vi "galvo.scan.engine_grMD.vi"() -> ()   [LabVIEW 2012]
doc: "SciScan 1.2 160622"
uses:
  <vilib>/Utility/VariantDataType/Type.ctl
  Custom Controls/trigger enum.ctl
  hyperscope modules/hyperscope subVIs/Timebase and Trigger Routing.ctl
  Custom Controls/advanced settings inner tab CTL.ctl
  GFG/GFGbooleanGet.vi
  GFG/GFGnumericGet.vi
  GFG/GFGstringGet.vi
  GFG/GFGfpRefGet.vi
  <vilib>/DAQmx/read.llb/DAQmx Read (Analog 2D I16 NChan NSamp).vi
  GFG/GFG library.lvlib
  <vilib>/Utility/VariantDataType/VariantType.lvlib
panel:
  out "String 3":string
  in  "stop":bool
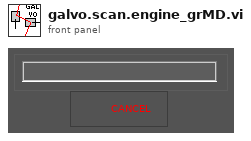
[diagram p1: front panel]
types:
  T1 = typedef "Timebase and Trigger Routing.ctl" = enum16{"Connect", "Disconnect all", "Disconnect Trigger"}
  T2 = typedef "trigger enum.ctl" = enum16{"legacy frame pulser PFI4", "continuous pulses", "single pulse", "trigger off"}
  T3 = enum32{"Invalid", "Default", "Floating", "Floating/Auto-Hide", "Modal"}
  T4 = enum32{"Invalid", "Standard", "Closed", "Hidden", "Minimized", "Maximized"}
  T5 = typedef "advanced settings inner tab CTL.ctl" = enum32{"arb. frames", "AO", "AI", "channels", "trigger", "Zstack data"}
  T6 = cluster{"NewVal":bool, "Event Registration Refnum":refnum<event-registration>}
  T7 = cluster{"WaveformChartRef":refnum<vi>, "DigitalRef":refnum<vi>, "ArrayRef":refnum<vi>, "TabControlRef":refnum<vi>, "EnumRef":refnum<vi>, "RingRef":refnum<vi>, "BooleanRef":refnum<vi>, "KnobRef":refnum<vi>, "SlideRef":refnum<vi>, "PathRef":refnum<vi>, "StringRef":refnum<vi>, "ComboBox":refnum<vi>, "WaveformGraphRef":refnum<vi>}
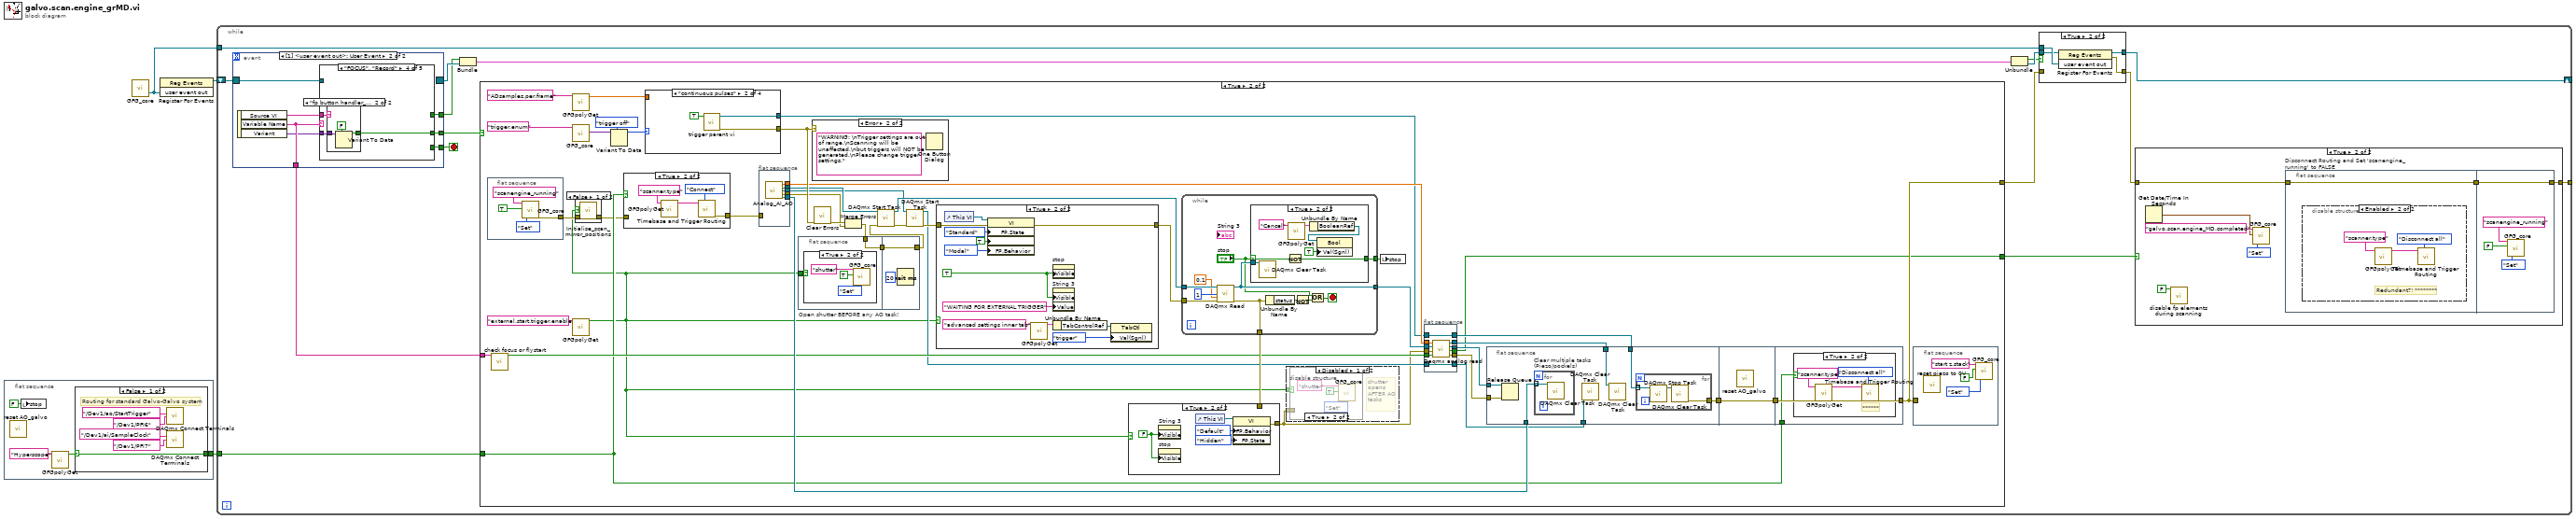
[diagram p0: block diagram]
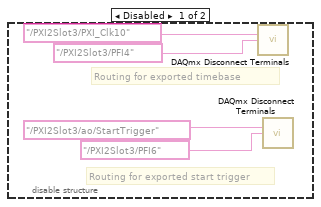
[diagram p5: hidden frame]
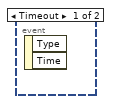
[diagram p6: hidden frame]
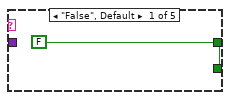
[diagram p7: hidden frame]
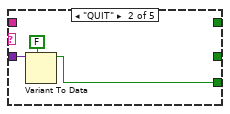
[diagram p8: hidden frame]
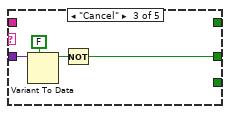
[diagram p9: hidden frame]
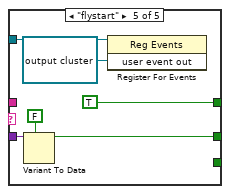
[diagram p11: hidden frame]
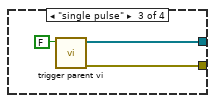
[diagram p20: hidden frame]
diagram:
  n1 = flat-sequence {
    tunnel: [w4] -> w1
    frame #0 {
      n2 = call "reset AO_galvo.vi"() -> ()  [unwired: 12 in]
      n3 = local write "stop"(FALSE ("stop")) -> ()
      n4 = call-poly "GFGpolyGet.vi"("Variable Name in"="Hyperscope") -> ("Boolean Value OUT"=w6:bool)  [unwired: 9 in, 1 out]
      n5 = case shown="False" w6 {
        selector: w6 -> [w9 w13]
        tunnel: [w9 w13] -> w4
        frame False {
          # "Routing for standard Galvo-Galvo system"
          n6 = call <vilib>:"DAQmx Connect Terminals.vi"("source terminal"=tag "/Dev1/ao/StartTrigger", "destination terminal"=tag "/Dev1/PFI6") -> ()  [unwired: 13 in, 1 out]
          n7 = call <vilib>:"DAQmx Connect Terminals.vi"("source terminal"=tag "/Dev1/ai/SampleClock", "destination terminal"=tag "/Dev1/PFI7") -> ()  [unwired: 13 in, 1 out]
        }
        frame True {
        }
      }
    }
  }
  n8 = call "GFG_core.vi"() -> ("user event out"=w2:refnum<user-event>)  [unwired: 13 in, 6 out]
  n9 = register-events(w2) -> (reference out=w3:refnum<event-registration>)  [unwired: 2 in, 1 out]
  n10 = while {
    tunnel: w2 -> [w26]
    shift-right: [w23] -> _
    shift-left: w3 -> [w27]
    tunnel: w1 -> [w16]
    tunnel: [w14] -> _
    stop <- w28 stop-if-true
    n11 = event shown="[1] <user event out>: User Event" {
      selector: w27 -> [_ w59]
      dyn-events: [_ _] -> w22
      timeout: _ -> [_ _]
      tunnel: [_ w62] -> w29
      tunnel: [_ w61] -> w28
      tunnel: [_ w58] -> w25
      tunnel: [_ w57] -> w21
      event Timeout {
        n12 = event-data() -> ()  [unwired: 1 in, 2 out]
      }
      event User Event {
        n13 = event-data() -> ("Source VI"=w60:string, "Variable Name"=w58:string, "Variant"=w56:variant)  [unwired: 1 in]
        n14 = case shown="\"FOCUS\", \"Record\"" w58 {
          tunnel: [w63 _ w67 w72 w80] -> w62
          tunnel: [w63 w64 _ _ _] -> w61
          tunnel: w56 -> [_ w66 w69 w73 w81]
          tunnel: w60 -> [_ _ _ w71 _]
          tunnel: w59 -> [_ _ _ _ w78]
          tunnel: [_ _ _ _ TRUE ("NewVal")] -> w57
          frame "False", Default {
            w63 = FALSE ("NewVal")
          }
          frame "QUIT" {
            n15 = Variant To Data(type=FALSE ("NewVal"), Variant=w66) -> (data=w64:bool)  [unwired: 1 in, 1 out]
          }
          frame "Cancel" {
            n16 = Variant To Data(type=FALSE ("NewVal"), Variant=w69) -> (data=w68:bool)  [unwired: 1 in, 1 out]
            n17 = Not(x=w68) -> (.not. x?=w67:bool)
          }
          frame "FOCUS", "Record" {
            n18 = case shown="\"fp button handler_crMD.vi\"" w71 {
              tunnel: w73 -> [_ w75]
              tunnel: [_ w74] -> w72
              frame "False", Default {
              }
              frame "fp button handler_crMD.vi" {
                n19 = Variant To Data(type=FALSE ("NewVal"), Variant=w75) -> (data=w74:bool)  [unwired: 1 in, 1 out]
              }
            }
          }
          frame "flystart" {
            n20 = Variant To Data(type=FALSE ("NewVal"), Variant=w81) -> (data=w80:bool)  [unwired: 1 in, 1 out]
            n21 = register-events(reference=w78, refnum<user-event> refnum ("user event out")) -> ()  [unwired: 1 in, 2 out]
          }
        }
      }
    }
    n22 = Bundle("NewVal"=w21, "Event Registration Refnum"=w22) -> (w20:T6)  [unwired: 1 in]
    n23 = case shown="True" w29 {
      tunnel: [_ w122] -> w24
      tunnel: w25 -> [_ w123]
      tunnel: [_ w95] -> w17
      tunnel: w16 -> [_ w90]
      frame False {
      }
      frame True {
        n24 = flat-sequence {
          tunnel: [w141] -> w85
          frame #0 {
            n25 = call "GFG_core.vi"("Variable Name in"="scanengine_running", "Variant in"=TRUE, "Action"=enum16{"Init", "Set", "Get"}."Set") -> ("error out"=w141:errorcluster)  [unwired: 10 in, 6 out]
          }
        }
        n26 = call "check focus or flystart.vi"("GFG variable name"=w123) -> ("Focus or flystart?"=w102:bool)  [unwired: 10 in]
        n27 = call-poly "GFGpolyGet.vi"("Variable Name in"="ADsamples.per.frame" ("Tag in")) -> ("Numeric"=w112:dbl)  [unwired: 8 in, 2 out]
        n28 = call "GFG_core.vi"("Variable Name in"="trigger.enum") -> ("Variant Out"=w118:variant)  [unwired: 12 in, 6 out]
        n29 = call-poly "GFGpolyGet.vi"("Variable Name in"="external.start.trigger.enable" ("Tag in")) -> ("Boolean Value OUT"=w83:bool)  [unwired: 9 in, 1 out]
        n30 = case shown="False" w83 {
          tunnel: w85 -> [w127 w128]
          tunnel: [w126 w128] -> w84
          frame False {
            n31 = call "Initialise_scan_mirror_positions.vi"("error in (no error)"=w127) -> ("error out"=w126:errorcluster)  [unwired: 10 in]
          }
          frame True {
          }
        }
        n32 = Variant To Data(type=trigger_enum."trigger off" ("trigger.enum"), Variant=w118) -> (data=w116:T2)  [unwired: 1 in, 1 out]
        n33 = case shown="True" w90 {
          tunnel: [_ w152] -> w91
          tunnel: w84 -> [_ _]
          frame False {
          }
          frame True {
            n34 = call-poly "GFGpolyGet.vi"("Variable Name in"="scanner.type") -> ("String"=w151:string)  [unwired: 9 in, 1 out]
            n35 = call "Timebase and Trigger Routing.vi"("Signal Router Action"=Timebase_and_Trigger_Routing."Connect", "System Type"=w151) -> ("error out"=w152:errorcluster)  [unwired: 9 in]
          }
        }
        n36 = case shown="\"continuous pulses\"" w116 {
          tunnel: [_ w166 w169 w171] -> w101
          tunnel: w112 -> [_ _ _ w172]
          tunnel: [_ w165 w168 _] -> w114
          frame Default {
          }
          frame "continuous pulses" {
            n37 = call "trigger parent vi.vi"("T=continuous, F=finite"=TRUE) -> ("error out"=w165:errorcluster, "ctr tasks out"=w166:refnum<k21>[])  [unwired: 9 in]
          }
          frame "single pulse" {
            n38 = call "trigger parent vi.vi"("T=continuous, F=finite"=FALSE) -> ("error out"=w168:errorcluster, "ctr tasks out"=w169:refnum<k21>[])  [unwired: 9 in]
          }
          frame "legacy frame pulser PFI4" {
            n39 = call "configure frame pulser.vi"("ADsamples.per.frame"=w172) -> ("frame pulser task out"=w173:refnum<k21>)  [unwired: 10 in]
            n40 = Build Array(w173) -> (w171:refnum<k21>[])
          }
        }
        n41 = flat-sequence {
          tunnel: [w149] -> w110
          tunnel: [w148] -> w109
          tunnel: [w147] -> w108
          tunnel: [w145] -> w107
          tunnel: [w146] -> w103
          tunnel: w91 -> [_]
          frame #0 {
            n42 = call "Analog_AI_AO.vi"() -> ("Timeout (s)"=w146:dbl, "Input task"=w149:refnum<k21>, "AO Output task"=w148:refnum<k21>, "error out"=w147:errorcluster, "Array of Piezo and Pockels Task"=w145:refnum<k21>[])  [unwired: 11 in]
          }
        }
        n43 = flat-sequence "Open shutter BEFORE any AO task!" {
          tunnel: w83 -> [w130]
          tunnel: w88 -> [w129]
          tunnel: [w129] -> w87
          tunnel: w87 -> [w134]
          tunnel: [w134] -> w86
          frame #0 {
            n44 = case shown="True" w130 {
              frame False {
                # "shutter already triggered in Config AI AO"
              }
              frame True {
                n45 = call "GFG_core.vi"("Variable Name in"="shutter" ("Tag in"), "Variant in"=TRUE, "Action"=enum16{"Init", "Set", "Get"}."Set") -> ()  [unwired: 10 in, 7 out]
              }
            }
          }
          frame #1 {
            n46 = Wait (ms)(milliseconds to wait=u32 20) -> ()  [unwired: 1 out]
          }
        }
        n47 = case shown="Error" w114 {
          frame No Error {
          }
          frame Error {
            n48 = One Button Dialog(message="WARNING: \nTrigger settings are out of range.\nScanning will be unaffected,\nbut triggers will NOT be generated.\nPlease change trigger settings.") -> ()  [unwired: 1 in, 1 out]
          }
        }
        n49 = call <vilib>:"Clear Errors.vi"("error in (no error)"=w114) -> ("error out"=w115:errorcluster)  [unwired: 6 in]
        n50 = Merge Errors(w115, w108) -> (w88:errorcluster)
        n51 = call <vilib>:"DAQmx Start Task.vi"("task/channels in"=w110, "error in"=w86) -> ("task out"=w124:refnum<k21>, "error out"=w125:errorcluster)  [unwired: 12 in]
        n52 = call <vilib>:"DAQmx Start Task.vi"("task/channels in"=w109, "error in"=w125) -> ("task out"=w97:refnum<k21>, "error out"=w106:errorcluster)  [unwired: 12 in]
        n53 = case shown="True" w83 {
          tunnel: [w197 w208] -> w105
          tunnel: w106 -> [w197 w199]
          frame False {
          }
          frame True {
            w206 = TRUE ("Visible")
            n54 = control-ref of="This VI"() -> (w200:refnum<vi>)
            n55 = property class="VI"(reference=w200, error in=w199, "FP.State"=T4."Standard" ("Front Panel Window:State"), "Front Panel.IsFrontmost"=TRUE ("Front Panel Window:Is Frontmost"), "FP.Behavior"=T3."Modal" ("Front Panel Window:Behavior")) -> (error out=w208:errorcluster)  [unwired: 1 out]
            n56 = call-poly "GFGpolyGet.vi"("Variable Name in"="advanced settings inner tab") -> ("output cluster"=w203:T7)  [unwired: 9 in, 1 out]
            n57 = property on="stop" class="Bool (strict)"("Visible"=w206) -> ()  [unwired: 2 in, 2 out]
            n58 = property on="String 3" class="Str"("Visible"=w206, "Value"="WAITING FOR EXTERNAL TRIGGER" ("String 3")) -> ()  [unwired: 2 in, 2 out]
            n59 = Unbundle By Name(w203) -> ("TabControlRef"=w198:refnum<vi>)
            n60 = property class="TabCtl"(reference=w198, "Val(Sgnl)"=advanced_settings_inner_tab_CTL."trigger" ("advanced settings inner tab")) -> ()  [unwired: 1 in, 2 out]
          }
        }
        n61 = while {
          tunnel: w105 -> [w220]
          tunnel: w124 -> [w219]
          tunnel: [w212] -> w104
          tunnel: [w215] -> w121
          tunnel: [w210] -> w120
          stop <- w214 stop-if-true
          n62 = call-poly <vilib>:"DAQmx Read.vi"("task/channels in"=w219, "number of samples per channel"=1, "timeout"=0.1, "error in"=w220) -> ("task out"=w212:refnum<k21>, "error out"=w215:errorcluster)  [unwired: 9 in, 1 out]
          n63 = case shown="True" "stop" {
            selector: "stop" -> [w221 w223]
            tunnel: w212 -> [_ w228]
            tunnel: [w221 w222] -> w210
            frame False {
            }
            frame True {
              n64 = call <vilib>:"DAQmx Clear Task.vi"("task in"=w228) -> ()  [unwired: 14 in, 1 out]
              n65 = Not(x=w223) -> (.not. x?=w222:bool)
              n66 = call-poly "GFGpolyGet.vi"("Variable Name in"="Cancel") -> ("output cluster"=w225:T7)  [unwired: 9 in, 1 out]
              n67 = Unbundle By Name(w225) -> ("BooleanRef"=w226:refnum<vi>)
              n68 = property class="Bool"(reference=w226, "Val(Sgnl)"=TRUE ("Visible")) -> ()  [unwired: 1 in, 2 out]
            }
          }
          n69 = Unbundle By Name(w215) -> ("status"=w216:bool)
          n70 = Not(x=w216) -> (.not. x?=w213:bool)
          n71 = Or(x="stop", y=w213) -> (x .or. y?=w214:bool)
        }
        n72 = case shown="True" w83 {
          tunnel: w121 -> [w191 _]
          tunnel: [w191 w196] -> w89
          frame False {
          }
          frame True {
            w195 = FALSE ("Visible")
            n73 = property on="String 3" class="Str"("Visible"=w195) -> ()  [unwired: 2 in, 2 out]
            n74 = property on="stop" class="Bool (strict)"("Visible"=w195) -> ()  [unwired: 2 in, 2 out]
            n75 = control-ref of="This VI"() -> (w192:refnum<vi>)
            n76 = property class="VI"(reference=w192, "FP.Behavior"=T3."Default" ("Front Panel Window:Behavior"), "FP.State"=T4."Hidden" ("Front Panel Window:State")) -> (error out=w196:errorcluster)  [unwired: 1 in, 1 out]
          }
        }
        n77 = disable-structure shown="Disabled" {
          disable-tunnel: w83 -> [w137 _]
          disable-tunnel: w89 -> [w136 _]
          frame Disabled {
            # "shutter opens AFTER AO tasks"
            n78 = case shown="True" w137 {
              tunnel: w136 -> [_ _]
              frame False {
              }
              frame True {
                n79 = call "GFG_core.vi"("Variable Name in"="shutter" ("Tag in"), "Variant in"=TRUE, "Action"=enum16{"Init", "Set", "Get"}."Set") -> ()  [unwired: 10 in, 7 out]
              }
            }
          }
          frame Enabled {
          }
        }
        n80 = local write "stop"(w120) -> ()
        n81 = flat-sequence {
          tunnel: w104 -> [w163]
          tunnel: w103 -> [w162]
          tunnel: w89 -> [w161]
          tunnel: w102 -> [w160]
          tunnel: w101 -> [w159]
          tunnel: [w159] -> w99
          tunnel: [w158] -> w100
          tunnel: [w157] -> w98
          tunnel: [w156] -> w94
          tunnel: w97 -> [w155]
          tunnel: [w155] -> w96
          tunnel: [w154] -> w95
          frame #0 {
            n82 = call "Daqmx analog read.vi"("Focus or flystart?"=w160, "error in"=w161, "task in"=w163, "Timeout (s)"=w162) -> ("error out"=w156:errorcluster, "DAQ loop terminated?"=w154:bool, "queue out"=w157:refnum<queue>, "task out"=w158:refnum<k21>)  [unwired: 4 in]
          }
        }
        n83 = flat-sequence {
          tunnel: w100 -> [w180]
          tunnel: w96 -> [w179]
          tunnel: w98 -> [w178]
          tunnel: w94 -> [w174]
          tunnel: w107 -> [w177]
          tunnel: w99 -> [w175]
          tunnel: [w176] -> w93
          tunnel: w93 -> [w185]
          tunnel: [w185] -> w92
          tunnel: [w187] -> w122
          tunnel: w92 -> [w187]
          tunnel: w90 -> [w186]
          frame #0 {
            n84 = Release Queue(queue=w178, error in (no error)=w174) -> ()  [unwired: 1 in, 3 out]
            n85 = for "Clear multiple tasks \n(Piezo/pockels)" {
              tunnel: w177 -> [w181] mode=indexing
              n86 = call <vilib>:"DAQmx Clear Task.vi"("task in"=w181) -> ()  [unwired: 14 in, 1 out]
            }
            n87 = call <vilib>:"DAQmx Clear Task.vi"("task in"=w179) -> ()  [unwired: 14 in, 1 out]
            n88 = call <vilib>:"DAQmx Clear Task.vi"("task in"=w180) -> ()  [unwired: 14 in, 1 out]
            n89 = for {
              tunnel: [w184] -> w176
              tunnel: w175 -> [w182] mode=indexing
              n90 = call <vilib>:"DAQmx Stop Task.vi"("task/channels in"=w182) -> ("task out"=w183:refnum<k21>)  [unwired: 13 in, 1 out]
              n91 = call <vilib>:"DAQmx Clear Task.vi"("task in"=w183) -> ("error out"=w184:errorcluster)  [unwired: 14 in]
            }
          }
          frame #1 {
            n92 = call "reset AO_galvo.vi"() -> ()  [unwired: 12 in]
          }
          frame #2 {
            n93 = case shown="True" w186 {
              frame False {
              }
              frame True {
                # "******"
                n94 = call-poly "GFGpolyGet.vi"("Variable Name in"="scanner.type") -> ("String"=w190:string)  [unwired: 9 in, 1 out]
                n95 = call "Timebase and Trigger Routing.vi"("Signal Router Action"=Timebase_and_Trigger_Routing."Disconnect all", "System Type"=w190) -> ()  [unwired: 9 in, 1 out]
              }
            }
          }
        }
        n96 = flat-sequence {
          tunnel: w122 -> [_]
          frame #0 {
            n97 = call "reset piezo to 0V.vi"() -> ()  [unwired: 11 in, 1 out]
            n98 = call "GFG_core.vi"("Variable Name in"="start z.stack", "Variant in"=FALSE ("Boolean"), "Action"=enum16{"Init", "Set", "Get"}."Set") -> ()  [unwired: 10 in, 7 out]
          }
        }
      }
    }
    n99 = Unbundle(w20) -> ("NewVal"=w18:bool, "Event Registration Refnum"=w19:refnum<event-registration>)
    n100 = case shown="True" w18 {
      tunnel: w26 -> [_ w35]
      tunnel: w24 -> [w30 _]
      tunnel: [w31 w34] -> w23
      tunnel: w19 -> [w31 w33]
      tunnel: [w30 w32] -> w15
      frame False {
      }
      frame True {
        n101 = register-events(reference=w33, w35) -> (reference out=w34:refnum<event-registration>, error out=w32:errorcluster)  [unwired: 1 in]
      }
    }
    n102 = case shown="True" w17 {
      tunnel: w15 -> [w36 w38]
      tunnel: [w36 w37] -> w14
      frame False {
      }
      frame True {
        n103 = Get Date/Time In Seconds() -> (seconds since 1Jan1904=w41:timestamp)
        n104 = call "disable fp elements during scanning.vi"("T for grey out"=FALSE) -> ()  [unwired: 11 in]
        n105 = call "GFG_core.vi"("Variable Name in"="galvo.scan.engine_MD.completed", "Variant in"=w41, "Action"=enum16{"Init", "Set", "Get"}."Set") -> ()  [unwired: 10 in, 7 out]
        n106 = flat-sequence "Disconnect Routing and Set 'scanengine_running' to FALSE" {
          tunnel: w38 -> [w44]
          tunnel: [w44] -> w39
          tunnel: w39 -> [w52]
          tunnel: [w52] -> w37
          frame #0 {
            n107 = disable-structure shown="Enabled" {
              frame Disabled {
                # "Routing for exported start trigger"
                # "Routing for exported timebase"
                n108 = call <vilib>:"DAQmx Disconnect Terminals.vi"("source terminal"=tag "/PXI2Slot3/PXI_Clk10", "destination terminal"=tag "/PXI2Slot3/PFI4") -> ()  [unwired: 13 in, 1 out]
                n109 = call <vilib>:"DAQmx Disconnect Terminals.vi"("source terminal"=tag "/PXI2Slot3/ao/StartTrigger", "destination terminal"=tag "/PXI2Slot3/PFI6") -> ()  [unwired: 13 in, 1 out]
              }
              frame Enabled {
                # "Redundant?! ********"
                n110 = call-poly "GFGpolyGet.vi"("Variable Name in"="scanner.type") -> ("String"=w50:string)  [unwired: 9 in, 1 out]
                n111 = call "Timebase and Trigger Routing.vi"("Signal Router Action"=Timebase_and_Trigger_Routing."Disconnect all", "System Type"=w50) -> ()  [unwired: 9 in, 1 out]
              }
            }
          }
          frame #1 {
            n112 = call "GFG_core.vi"("Variable Name in"="scanengine_running", "Variant in"=FALSE, "Action"=enum16{"Init", "Set", "Get"}."Set") -> ()  [unwired: 10 in, 7 out]
          }
        }
      }
    }
  }
